vi "Start_Stop_Tasks.vi"(8 "error in":errorcluster, 10 "Start/Stop Task":bool, 11 "Tasks In":refnum<k21>[](array[refnum])) -> (0 "error out":errorcluster, 2 "error?":bool, 3 "Tasks Out":refnum<k21>[](array[refnum]))   [LabVIEW 2025, in "Control.lvlib"]
uses:
  Control/Control.lvlib
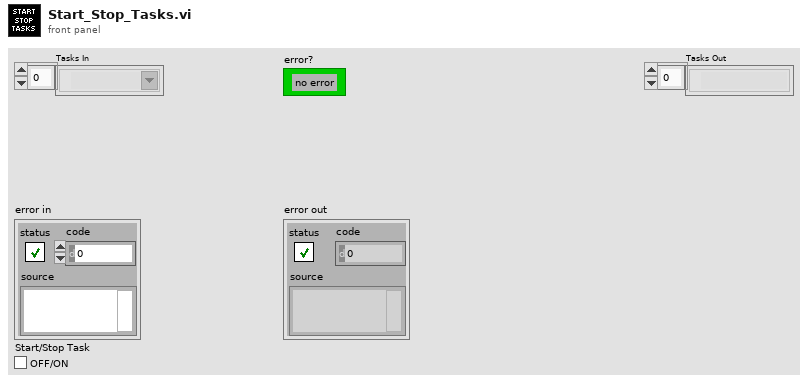
[diagram p1: front panel]
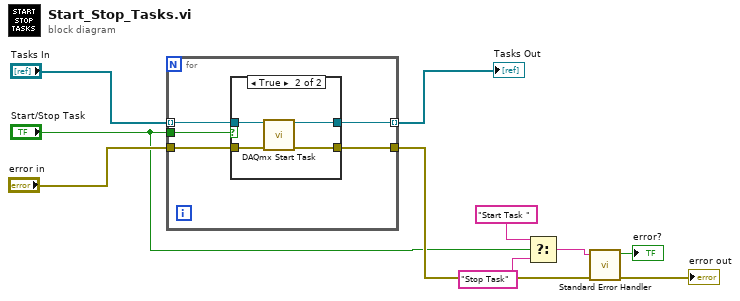
[diagram p0: block diagram]
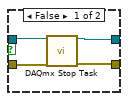
[diagram p2: hidden frame]
diagram:
  n1 = for {
    tunnel: "Tasks In" -> [w15] mode=indexing
    tunnel: "error in" -> [w14]
    tunnel: [w13] -> w8
    tunnel: [w12] -> w9 mode=indexing
    tunnel: "Start/Stop Task" -> [w11]
    n2 = case shown="True" w11 {
      tunnel: w15 -> [w19 w23]
      tunnel: w14 -> [w18 w22]
      tunnel: [w17 w21] -> w13
      tunnel: [w16 w20] -> w12
      frame False {
        n3 = call <vilib>:"DAQmx Stop Task.vi"("task/channels in"=w19, "error in"=w18) -> ("task out"=w16:refnum<k21>, "error out"=w17:errorcluster)  [unwired: 12 in]
      }
      frame True {
        n4 = call <vilib>:"DAQmx Start Task.vi"("task/channels in"=w23, "error in"=w22) -> ("task out"=w20:refnum<k21>, "error out"=w21:errorcluster)  [unwired: 12 in]
      }
    }
  }
  "Tasks Out" <- w9
  n5 = Select(t="Start Task " ("source"), s="Start/Stop Task", f="Stop Task") -> (s? t:f=w5:string)
  n6 = call "Standard Error Handler.vi"("error in (no error)"=w8, "source"=w5) -> ("error out"=→"error out":errorcluster, "error?"=→"error?":bool)  [unwired: 8 in]
